vi "Main.vi"() -> ()   [LabVIEW 2018]
uses:
  <vilib>/addons/database/Connection.llb/DB Tools Open Connec (String).vi
  <vilib>/addons/database/NI_Database_API.lvlib
  <vilib>/ptbypt/NI_PtbyPt.lvlib
panel:
  out "100看门狗 2":i32
  in  "90数据":string[](array[string])
  in  "70数据":string[](array[string])
  out "Code":string
  in  "扫描到的条码":string
  in  "打印的条码":string
  out "退出":bool
  out "Main Tab":T1(tab)
  out "产品型号10":string
  out "产品型号20-90":string
  in  "其它信息":enum32{"信息", "错误信息"}(tab)
  out "ST20通讯状态":bool caption="ST30通讯状态"
  in  "ST100产品类型":string
  in  "ST100操作者":string
  in  "ST90产品类型":string
  in  "ST90操作者":string
  in  "ST80产品类型":string
  in  "ST80操作者":string
  in  "ST70产品类型":string
  in  "ST70操作者":string
  in  "ST60产品类型":string
  in  "ST60操作者":string
  in  "ST50产品类型":string
  in  "ST50操作者":string
  in  "ST40产品类型":string
  in  "ST40操作者":string
  in  "ST30产品类型":string
  in  "ST30操作者":string
  in  "ST20产品类型":string
  in  "ST20操作者":string
  in  "ST10产品类型":string
  in  "ST10操作者":string
  out "ST10通讯状态":bool
  out "ST30通讯状态":bool
  out "ST40通讯状态":bool caption="ST30通讯状态"
  out "ST70通讯状态":bool caption="ST30通讯状态"
  out "ST50通讯状态":bool caption="ST30通讯状态"
  out "ST60通讯状态":bool caption="ST30通讯状态"
  out "ST80通讯状态":bool caption="ST30通讯状态"
  out "ST90通讯状态":bool caption="ST30通讯状态"
  out "ST100通讯状态":bool caption="ST30通讯状态"
  in  "错误信息":i32(listbox)
  in  "每工站主要显示":T2(tab)
  in  "ST102_DATA":i32(listbox)=7 caption="ST10_DATA"
  in  "ST101_DATA":i32(listbox)=9 caption="ST10_DATA"
  out "ST10曲线":cluster{"X":dbl, "Y":dbl}[](graph) caption="ST20曲线"
  in  "选项卡控件":enum32{"数据", "曲线"}(tab)
  in  "ST202_DATA":i32(listbox) caption="ST20_DATA"
  in  "ST201_DATA":i32(listbox) caption="ST20_DATA"
  out "ST201_R曲线":cluster{"X":dbl, "Y":dbl}[](graph) caption="ST20曲线"
  out "ST202曲线":cluster{"X":dbl, "Y":dbl}[](graph) caption="ST20曲线"
  out "ST201_L曲线":cluster{"X":dbl, "Y":dbl}[](graph) caption="ST20曲线"
  in  "ST303_DATA":i32(listbox) caption="ST30_DATA"
  in  "ST302_DATA":i32(listbox) caption="ST30_DATA"
  in  "ST301_DATA":i32(listbox) caption="ST30_DATA"
  in  "ST402_DATA":i32(listbox) caption="ST40_DATA"
  in  "ST401_DATA":i32(listbox) caption="ST40_DATA"
  in  "选项卡控件 2":enum32{"数据1", "数据2", "曲线"}(tab)
  in  "ST502_DATA":i32(listbox)=4 caption="ST50_DATA"
  in  "ST501_DATA":i32(listbox)=4 caption="ST50_DATA"
  in  "ST504_DATA":i32(listbox)=4 caption="ST50_DATA"
  in  "ST503_DATA":i32(listbox)=4 caption="ST50_DATA"
  out "ST50_R曲线":cluster{"X":dbl, "Y":dbl}[](graph) caption="ST20曲线"
  out "ST50_L曲线":cluster{"X":dbl, "Y":dbl}[](graph) caption="ST20曲线"
  in  "ST603_DATA":i32(listbox) caption="ST60_DATA"
  in  "ST602_DATA":i32(listbox) caption="ST60_DATA"
  in  "ST601_DATA":i32(listbox) caption="ST60_DATA"
  in  "选项卡控件 3":enum32{"数据", "曲线"}(tab)
  in  "ST70_DATA":i32(listbox)=2
  out "ST70_R曲线":cluster{"X":dbl, "Y":dbl}[](graph) caption="ST20曲线"
  out "ST70_L曲线":cluster{"X":dbl, "Y":dbl}[](graph) caption="ST20曲线"
  in  "ST80_DATA":i32(listbox)
  in  "ST901_DATA":i32(listbox) caption="ST80_DATA"
  in  "ST902_DATA":i32(listbox) caption="ST80_DATA"
  in  "登录界面":bool
  in  "注销":bool
  in  "修改密码":bool
  in  "Rework界面":bool
  in  "界面切换":bool
  in  "登录界面返回":bool
  out "登录状态":string
  in  "登录":bool
  in  "输入管理员密码":string
  in  "修改密码界面返回":bool
  out "修改密码状态":string
  in  "确认修改密码":bool
  in  "新密码":string
  in  "初始密码":string
  in  "603":bool
  in  "602":bool
  in  "504":bool
  in  "402":bool
  in  "303":bool
  in  "302":bool
  in  "202":bool
  out "Rework状态":string
  in  "查询":bool
  in  "确定Rework":bool
  in  "Rework返回":bool
  in  "输入需要Rework的一维码：":string
  in  "102":bool
  in  "201":bool
  in  "301":bool
  in  "401":bool
  in  "501":bool
  in  "502":bool
  in  "503":bool
  in  "601":bool
  in  "70":bool
  in  "80":bool
  in  "901":bool
  in  "902":bool
  in  "Monitor Tab":T3(tab)
  out "产品型号":u32
  out "画曲线T-201 2":u32
  out "ST201文件移动中":bool caption="ST201保存中"
  out "ST201保存中":bool
  out "ST10画曲线":bool
  in  "303数据回复输入":bool
  in  "303扫码回复输入":bool
  out "数据保存请求回复303":string
  out "上一站号 (303)":string
  out "上一站结果 (303)":string
  out "扫码请求回复303":string
  out "303二维码":string
  out "ST303数据读取":bool
  out "ST303扫码请求":bool
  out "ST303数据读取 (事件)":bool
  out "ST303扫码请求 (事件)":bool
  in  "302数据回复输入":bool
  in  "302扫码回复输入":bool
  out "数据保存请求回复302":string
  out "上一站号 (302)":string
  out "上一站结果 (302)":string
  out "扫码请求回复302":string
  out "302二维码":string
  out "ST302数据读取":bool
  out "ST302扫码请求":bool
  out "ST302数据读取 (事件)":bool
  out "ST302扫码请求 (事件)":bool
  in  "301数据回复输入":bool
  in  "301扫码回复输入":bool
  out "ST202数据保存请求":bool
  out "ST202扫码请求":bool
  out "ST201数据保存请求":bool
  out "上一站结果 (202)":string
  out "上一站号 (202)":string
  in  "102数据回复写入":bool
  in  "102扫码回复写入":bool
  out "ST202扫码请求(事件)":bool
  out "ST202画曲线":bool
  out "ST202数据读取(事件)":bool
  out "ST201画曲线":bool
  out "ST201数据读取(事件)":bool
  out "ST201扫码请求(事件)":bool
  out "数据保存请求回复102":string
  out "扫码请求回复102":string
  out "上一站结果(10)":string
  out "上一站号(10)":string
  out "ST102扫码请求":bool
  out "ST101扫码请求":bool
  out "ST102数据读取":bool
  out "扫码请求回复101":string
  out "ST102扫码请求（事件）":bool
  out "ST101扫码请求（事件）":bool
  out "ST102数据读取（事件）":bool
  out "101二维码":string caption="101 二维码"
  out "ST201扫码请求":bool
  out "数据保存请求回复201":string
  out "扫码请求回复201":string
  out "上一站结果 (201)":string
  out "上一站号 (201)":string
  out "201二维码":string
  in  "返回":bool
  out "Sleeve_5020001":string
  out "20看门狗":i32
  out "10看门狗":i32
  out "Flange_5025570":string
  out "202二维码":string
  out "扫码请求回复202":string
  out "101打码等级":string
  out "102二维码":string caption="102 二维码"
  out "ST102数据":string[](array[string])
  in  "101扫码回复写入":bool
  in  "201扫码回复写入":bool
  in  "202扫码回复写入":bool
  in  "202数据回复写入":bool
  out "数据保存请求回复202":string
  in  "201数据回复写入":bool
  out "201数据":string[](array[string])
  out "202data":string[](array[string])
  out "30看门狗":i32
  out "数据保存请求回复301":string
  out "上一站号 (301)":string
  out "上一站结果 (301)":string
  out "扫码请求回复301":string
  out "301二维码":string
  out "ST301数据读取":bool
  out "ST301扫码请求":bool
  out "ST301数据读取 (事件)":bool
  out "ST301扫码请求 (事件)":bool
  out "301数据":string[](array[string])
  out "302data":string[](array[string])
  out "303data":string[](array[string])
  out "OP201文件?":bool
  out "画曲线T--201":u32
  out "打开时间":u32
  out "ST502画曲线":bool
  out "504data":string[](array[string])
  out "上一站号 (504)":string
  out "上一站结果 (504)":string
  out "数据保存请求回复504":string
  out "扫码请求回复504":string
  out "ST504数据读取（事件）":bool
  out "ST504扫码请求（事件）":bool
  out "ST504数据读取":bool
  out "ST504扫码请求":bool
  out "504二维码":string
  in  "504数据回复输入":bool
  in  "504扫码回复输入":bool
  out "上一站号 (503)":string
  out "上一站结果 (503)":string
  out "数据保存请求回复503":string
  out "扫码请求回复503":string
  out "ST503数据读取（事件）":bool
  out "ST503扫码请求（事件）":bool
  out "上一站号 (502)":string
  out "上一站结果 (502)":string
  out "数据保存请求回复502":string
  out "扫码请求回复502":string
  out "ST502数据读取（事件）":bool
  out "ST502扫码请求（事件）":bool
  out "上一站号 (501)":string
  out "上一站结果 (501)":string
  out "数据保存请求回复501":string
  out "扫码请求回复501":string
  out "ST501数据读取（事件）":bool
  out "ST501扫码请求（事件）":bool
  out "ST401数据保存请求":bool
  out "ST401扫码请求":bool
  out "ST401数据读取（事件）":bool caption="ST401数据保存请求（事件）"
  out "ST401扫码请求（事件）":bool
  out "数据保存请求回复401":string
  out "扫码请求回复401":string
  out "401二维码":string
  in  "401数据回复写入":bool
  in  "401扫码回复写入":bool
  out "上一站号 (401)":string
  out "上一站结果 (401)":string
  out "ST402数据保存请求":bool
  out "ST402扫码请求":bool
  out "402data":string[](array[string])
  out "402二维码":string
  out "401数据":string[](array[string])
  out "40看门狗":i32
  in  "402扫码回复写入":bool
  in  "402数据回复写入":bool
  out "ST402数据读取（事件）":bool caption="ST402数据保存请求（事件）"
  out "ST402扫码请求（事件）":bool
  out "上一站号 (402)":string
  out "上一站结果 (402)":string
  out "数据保存请求回复402":string
  out "扫码请求回复402":string
  out "503data":string[](array[string])
  out "503二维码":string
  out "ST503数据读取":bool
  out "ST503扫码请求":bool
  out "ST502数据读取":bool
  out "ST502扫码请求":bool
  out "ST501数据读取":bool
  out "ST501扫码请求":bool
  out "502二维码":string
  out "501二维码":string
  in  "503数据回复输入":bool
  in  "503扫码回复输入":bool
  in  "502数据回复输入":bool
  in  "502扫码回复输入":bool
  in  "501数据回复输入":bool
  in  "501扫码回复输入":bool
  out "50看门狗":i32
  out "501data":string[](array[string])
  out "502数据":string[](array[string])
  out "ST70画曲线":bool
  out "上一站结果 (80)":string
  out "上一站号 (80)":string
  out "扫码请求回复80":string
  out "数据保存请求回复80":string
  out "ST80数据保存请求（事件）":bool
  out "ST80扫码请求 （事件）":bool caption="ST80扫码请求（事件）"
  out "数据保存请求回复70":string
  out "ST70数据读取（事件）":bool caption="ST70数据读取(事件)"
  out "上一站结果 (603)":string
  out "上一站号 (603)":string
  out "扫码请求回复603":string
  out "数据保存请求回复603":string
  out "ST603数据读取（事件）":bool
  out "ST603扫码请求（事件）":bool
  out "上一站结果 (602)":string
  out "上一站号 (602)":string
  out "扫码请求回复602":string
  out "数据保存请求回复602":string
  out "ST602数据读取（事件）":bool
  out "ST602扫码请求 （事件）":bool caption="ST602扫码请求（事件）"
  out "ST601数据读取（事件）":bool
  out "ST601扫码请求（事件）":bool
  out "603data":string[](array[string])
  out "603二维码":string
  out "ST603数据读取":bool
  out "ST603扫码请求":bool
  out "ST602数据读取":bool
  out "ST602扫码请求":bool
  out "ST601数据读取":bool
  out "ST601扫码请求":bool
  out "602data":string[](array[string])
  out "602二维码":string
  out "601数据":string[](array[string])
  out "601二维码":string
  in  "603数据回复输入":bool
  in  "603扫码回复输入":bool
  in  "602数据回复输入":bool
  in  "602扫码回复输入":bool
  in  "601数据回复输入":bool
  in  "601扫码回复输入":bool
  out "60看门狗":i32
  out "扫码请求回复601":string
  out "数据保存请求回复601":string
  out "上一站结果 (601)":string
  out "上一站号 (601)":string
  out "ST70数据读取":bool
  out "70编码":string
  in  "70数据回复输入":bool
  out "70看门狗":i32
  out "70数据":string[](array[string])
  out "ST70_Housing_5025351":string
  out "ST70_Bushing_5025400":string
  out "ST80数据保存请求":bool
  out "ST80扫码请求":bool
  out "80二维码":string
  in  "80数据回复写入":bool
  in  "80扫码回复写入":bool
  out "ST80_Spring_5024883":string
  out "ST80_Flat_sael_5020064":string
  out "ST80_Spring_plate_5025473":string
  out "80看门狗":i32
  out "80数据":string[](array[string])
  in  "ST70数据读取（事件） 2":bool caption="ST70数据读取(手动事件)"
  in  "70数据 2-手动测试":string[](array[string])
  out "ST90画曲线":bool
  in  "901数据回复输入":bool
  out "上一站号 (901)":string
  out "上一站结果 (901)":string
  out "数据保存请求回复901":string
  out "扫码请求回复901":string
  in  "901扫码回复输入":bool
  out "901二维码":string
  out "ST901扫码请求":bool
  out "ST901数据读取":bool
  out "ST901扫码请求（事件）":bool
  out "ST901数据读取（事件）":bool
  in  "901编码回复输入":bool
  out "901编码":string
  out "ST901编码请求":bool
  out "ST901编码请求 （事件）":bool caption="ST901编码请求（事件）"
  out "编码请求回复901":string
  out "上一站号 (901) 编码":string caption="上一站号 (901编码)"
  out "上一站结果 (901)编码":string caption="上一站结果 (901编码)"
  in  "902扫码回复输入":bool
  in  "902数据回复输入":bool
  out "ST902扫码请求":bool
  out "ST902数据读取":bool
  out "902二维码":string
  out "ST902扫码请求（事件）":bool
  out "ST902数据读取（事件）":bool
  out "数据保存请求回复902":string
  out "扫码请求回复902":string
  out "上一站号 (902)":string
  out "上一站结果 (902)":string
  out "901数据":string[](array[string])
  out "902数据":string[](array[string])
  out "90看门狗":i32
  out "ST100扫码请求":bool
  out "ST100扫码请求（事件）":bool
  out "上一站结果 (100)":string
  out "上一站号 (100)":string
  out "100二维码":string
  in  "100扫码回复输入":bool
  out "100看门狗":i32
  out "扫码请求回复100":string
  out "压机旋铆位移压力图_4":cluster{dbl[], dbl[]}(graph)
  out "压机旋铆位移压力图_3":cluster{dbl[], dbl[]}(graph)
  out "压机旋铆位移压力图_2":cluster{dbl[], dbl[]}(graph)
  out "压机旋铆位移压力图_1":cluster{dbl[], dbl[]}(graph)
  out "压机旋铆位移压力图_5":cluster{dbl[], dbl[]}(graph)
  # "V1.0"
  # "数据库追溯系统"
  # "v3.0"
  # "登 录"
  # "修 改 密 码"
  # "ST30"
  # "ST10"
  # "ST20"
  # "ST60"
  # "ST70"
  # "ST80"
  # "ST100"
  # "ST90"
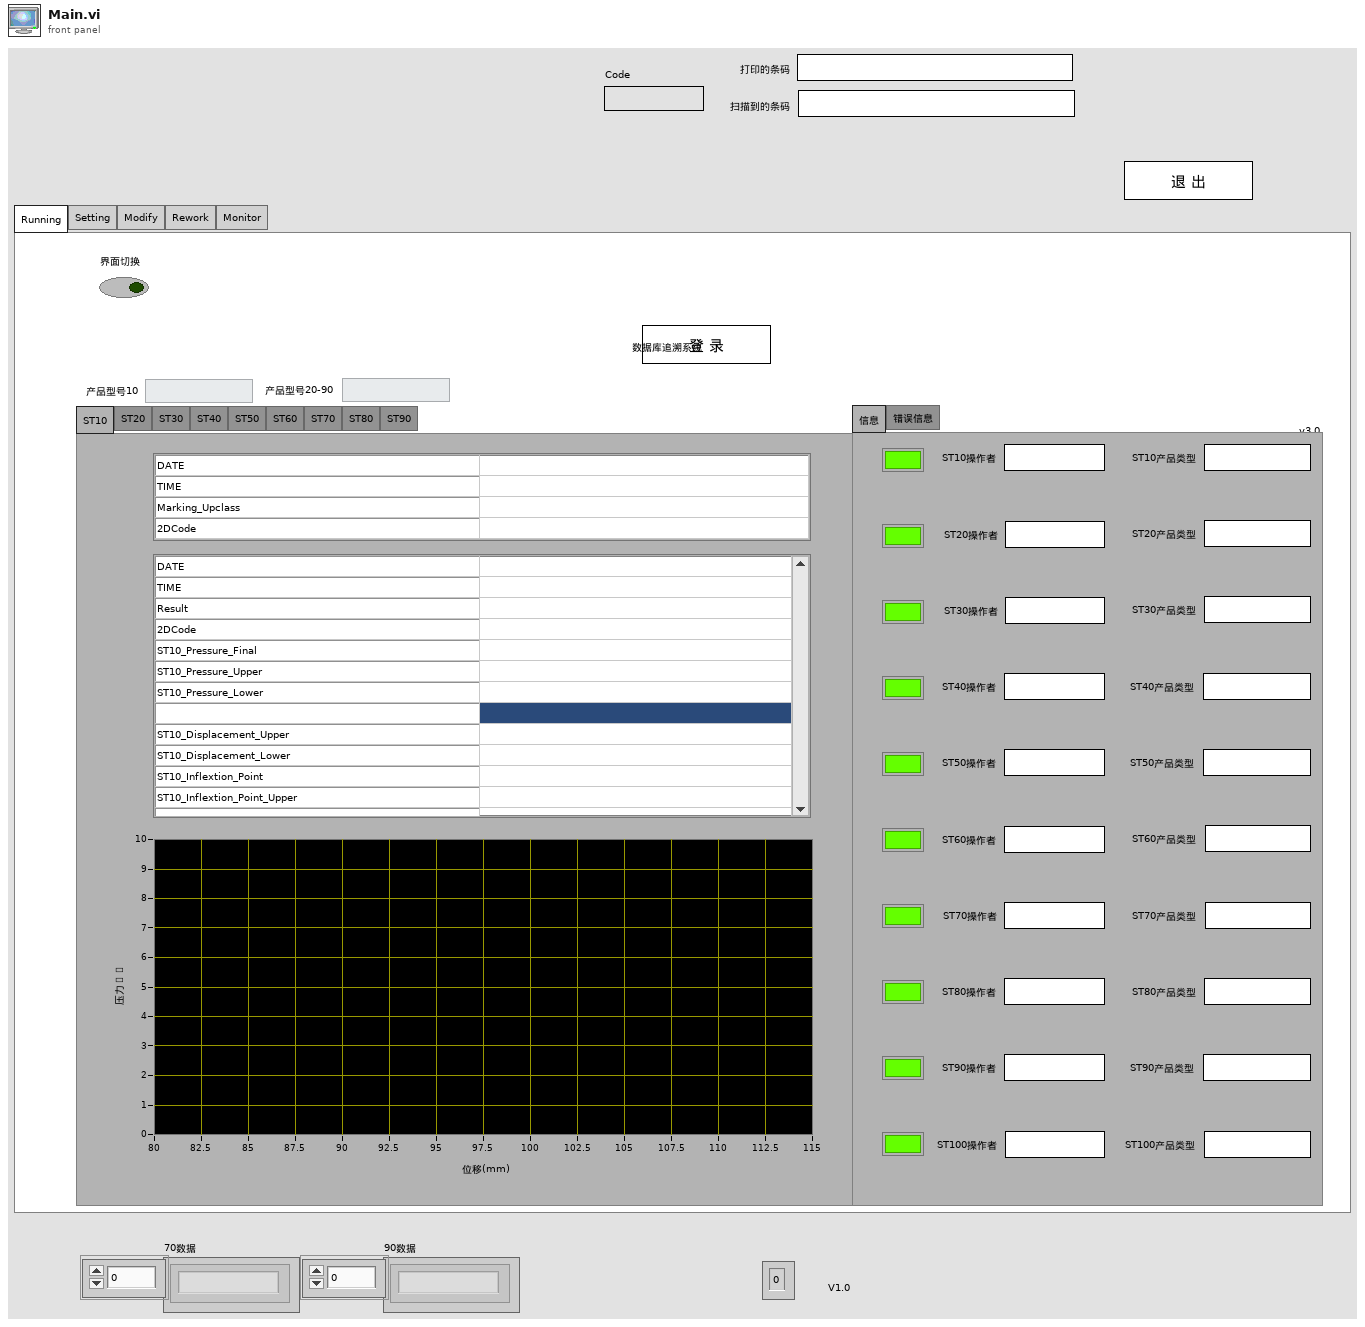
[diagram p1: front panel]
types:
  T1 = enum32{"Running", "Setting", "Modify", "Rework", "Monitor"}
  T2 = enum32{"ST10", "ST20", "ST30", "ST40", "ST50", "ST60", "ST70", "ST80", "ST90"}
  T3 = enum32{"Interface 1", "Interface 2", "Interface 3", "Interface 4", "Interface 7", "Interface 8"}
  T4 = enum32{"Invalid", "Standard", "Closed", "Hidden", "Minimized", "Maximized"}
  T5 = typedef "NI_Database_API.lvlib/Conn ObjectReference.ctl" = refnum<k1>
diagram:
  n1 = flat-sequence {
    tunnel: [w9] -> w2
    tunnel: [w8] -> w1
    tunnel: w2 -> [w35]
    tunnel: w1 -> [w36]
    frame #0 {
      w6 = "Code" ("subkeyName")
      w4 = FALSE ("可见")
      n2 = call "Read Registry.vi"("value"=w6, "subkeyName"=w6) -> ("Data"=→"Code":string)  [unwired: 6 in, 1 out]
      n3 = property on="Rework界面" class="Bool"("Visible"=w4) -> ()  [unwired: 2 in, 2 out]
      n4 = property on="注销" class="Bool"("Visible"=w4) -> ()  [unwired: 2 in, 2 out]
      n5 = property on="修改密码" class="Bool"("Visible"=w4) -> ()  [unwired: 2 in, 2 out]
      n6 = property on="界面切换" class="Bool (严格)"("Visible"=FALSE ("可见")) -> ()  [unwired: 2 in, 2 out]
      n7 = call-poly <vilib>:"DB Tools Open Connection.vi"("connection information"="DQ501") -> ("error out"=w8:errorcluster, "connection reference"=w9:T5)  [unwired: 7 in]
    }
    frame #1 {
      # "10\n201\n202\n50\n70"
      # "字符串的初始地址都加2位"
      # "报警日志 ：Alarm_Log\n历史程序：History program\n数据保存：data storage\n曲线curve\n数据data"
      # "报警日志 ：Alarm_Log\n历史程序：History program\n数据保存：data storage\n曲线curve\n数据data"
      # "报警日志 ：Alarm_Log\n历史程序：History program\n数据保存：data storage\n曲线curve\n数据data"
      # "报警日志 ：Alarm_Log\n历史程序：History program\n数据保存：data storage\n曲线curve\n数据data"
      # "报警日志 ：Alarm_Log\n历史程序：History program\n数据保存：data storage\n曲线curve\n数据data"
      # "对数据库操作的事件"
      # "其余事件 如曲线保存"
      n8 = constructor class="CloseExcel"() -> (reference out=w14:refnum<k24>, error out=w12:errorcluster)  [unwired: 3 in, 1 out]
      n9 = invoke class="CloseExcel" method="OpenProgram"(reference=w14, error in=w12) -> (reference out=w13:refnum<k24>, error out=w11:errorcluster)  [unwired: 1 in, 1 out]
      n10 = case shown="错误" w11 {
        selector: w11 -> [_ w40]
        tunnel: "CloseExcel进程打开失败！" -> [_ w43]
        frame No Error {
        }
        frame Error {
          n11 = property on="错误信息" class="LstBox (严格)"() -> ("Item Names"=w38:string[])  [unwired: 2 in, 2 out]
          n12 = Unbundle By Name(w40) -> ("source"=w39:string)
          n13 = Format Date/Time String(time format string (%c)="%Y-%m-%d %H:%M:%S" ("时间格式字符串(%c)")) -> (date/time string=w45:string)  [unwired: 2 in]
          n14 = Concatenate Strings(w45, "  " ("字符串"), w43, w39) -> (w41:string)
          n15 = Insert Into Array(array=w38, index=0 ("索引"), new element=w41) -> (w37:string[])
          n16 = property on="错误信息" class="LstBox (严格)"("Item Names"=w37) -> ()  [unwired: 2 in, 2 out]
        }
      }
      n17 = while {
        tunnel: w36 -> [w7757]
        tunnel: w35 -> [w7756]
        tunnel: w13 -> [w7755]
        stop <- w7759 stop-if-true
        n18 = event shown="[9] \"注销\": 值改变" {
          selector: _ -> [_ _ _ _ _ _ _ _ _ _ _ _ _ _ _ _ _ _]
          dyn-events: _ -> [_ _ _ _ _ _ _ _ _ _ _ _ _ _ _ _ _ _]
          timeout: 10 -> [_ _ _ _ _ _ _ _ _ _ _ _ _ _ _ _ _ _]
          tunnel: [FALSE TRUE FALSE FALSE FALSE FALSE FALSE FALSE FALSE FALSE FALSE FALSE FALSE FALSE _ FALSE _ _] -> w7759
          tunnel: w7757 -> [_ w7766 _ _ _ _ _ _ _ _ _ _ _ _ _ _ _ _]
          tunnel: w7756 -> [_ w7765 _ _ _ _ _ _ _ _ _ _ _ _ _ _ _ _]
          tunnel: w7755 -> [_ w7762 _ _ _ _ _ _ _ _ _ _ _ _ _ _ _ _]
          event Timeout {
            n19 = event-data() -> ()  [unwired: 1 in, 3 out]
          }
          event Panel Close {
            n20 = event-data() -> ()  [unwired: 1 in, 3 out]
            n21 = invoke class="CloseExcel" method="CloseProgram"(reference=w7762) -> ()  [unwired: 2 in, 3 out]
            n22 = call <vilib>:"DB Tools Close Connection.vi"("error in (no error)"=w7766, "connection reference"=w7765) -> ()  [unwired: 5 in, 1 out]
            n23 = flat-sequence {
              frame #0 {
                n24 = property on="错误信息" class="LstBox (严格)"() -> ("Item Names"=w7769:string[])  [unwired: 2 in, 2 out]
                n25 = Array Size(array=w7769) -> (size(s)=w7768:i32)
                n26 = Equal To 0?(x=w7768) -> (x = 0?=w7767:bool)
                n27 = case shown="假" w7767 {
                  tunnel: w7769 -> [w7770 _]
                  frame False {
                    n28 = call <vilib>:"Check if File or Folder Exists.vi"("path"=path "D:/Alarm_Log") -> ("error out"=w7786:errorcluster, "file or folder exists?"=w7787:bool, "dup path"=w7785:path)  [unwired: 8 in]
                    n29 = Format Date/Time String(time format string (%c)="%Y%m%d" ("时间格式字符串(%c)")) -> (date/time string=w7782:string)  [unwired: 2 in]
                    n30 = case shown="真" w7787 {
                      tunnel: w7786 -> [w7802 w7803]
                      tunnel: w7785 -> [w7801 w7804]
                      tunnel: [w7800 w7804] -> w7784
                      tunnel: [w7799 w7803] -> w7779
                      frame False {
                        n31 = Create Folder(path (use dialog)=w7801, error in=w7802) -> (created path=w7800:path, error out=w7799:errorcluster)  [unwired: 1 in, 1 out]
                      }
                      frame True {
                      }
                    }
                    n32 = Concatenate Strings(w7782, ".txt" ("字符串")) -> (w7780:string)
                    n33 = Build Path(base path=w7784, name or relative path=w7780) -> (appended path=w7773:path)
                    n34 = call <vilib>:"Check if File or Folder Exists.vi"("error in (no error)"=w7779, "path"=w7773) -> ("error out"=w7777:errorcluster, "file or folder exists?"=w7778:bool, "dup path"=w7776:path)  [unwired: 7 in]
                    n35 = case shown="假" w7778 {
                      tunnel: w7777 -> [_ w7792]
                      tunnel: w7776 -> [_ w7791]
                      tunnel: [string[] [] ("array of strings") w7790] -> w7774
                      frame False {
                      }
                      frame True {
                        n36 = Read from Text File(file (use dialog)=w7791, error in=w7792) -> (text=w7793:string)  [unwired: 2 in, 3 out]
                        n37 = Search and Replace String(replace all?=TRUE ("替换全部？(F)"), input string=w7793, search string="\n" ("搜索字符串"), replace string="\\" ("替换字符串(\"\")")) -> (result string=w7797:string)  [unwired: 4 in, 3 out]
                        n38 = String To Path(string=w7797) -> (path=w7798:path)
                        n39 = Path to Array of Strings(0:w7798) -> (2:w7790:string[])  [unwired: 1 out]
                      }
                    }
                    n40 = Array Size(array=w7770) -> (size(s)=w7775:i32)
                    n41 = Insert Into Array(array=w7770, index=w7775, new element=w7774) -> (w7772:string[])
                    n42 = Write to Text File(file (use dialog)=w7773, text=w7772) -> (error out=w7771:errorcluster)  [unwired: 2 in, 2 out]
                    n43 = call <vilib>:"Clear Errors.vi"("error in (no error)"=w7771) -> ()  [unwired: 5 in, 2 out]
                  }
                  frame True {
                  }
                }
              }
              frame #1 {
                n44 = control-ref of="本VI"() -> (w7805:refnum<vi>)
                n45 = property class="VI"(reference=w7805, "FP.State"=T4."Closed" ("前面板窗口:状态")) -> ()  [unwired: 1 in, 2 out]
              }
            }
            "退出" <- TRUE ("退出")
          }
          event "界面切换": Value Change {
            n46 = event-data() -> ()  [unwired: 1 in, 3 out]
            "Main Tab" <- T1."Monitor" ("Main Tab")
          }
          event "返回": Value Change {
            n47 = event-data() -> ()  [unwired: 1 in, 3 out]
            n48 = local write "Main Tab"(T1."Running" ("Main Tab")) -> ()
          }
          event "登录界面": Value Change {
            w7811 = "" ("输入管理员密码")
            n49 = event-data() -> ()  [unwired: 1 in, 3 out]
            n50 = local write "登录状态"(w7811) -> ()
            n51 = local write "输入管理员密码"(w7811) -> ()
            n52 = local write "Main Tab"(T1."Setting" ("Main Tab")) -> ()
          }
          event "登录": Value Change {
            n53 = event-data() -> ()  [unwired: 1 in, 3 out]
            n54 = Equal?(x="输入管理员密码", y="18202173350") -> (x = y?=w7814:bool)
            n55 = case shown="真" w7814 {
              tunnel: "输入管理员密码" -> [w7825 _]
              tunnel: [w7824 TRUE] -> w7815
              frame False {
                n56 = local read "Code"() -> (w7826:string)
                n57 = Equal?(x=w7825, y=w7826) -> (x = y?=w7824:bool)
              }
              frame True {
                n58 = property on="界面切换" class="Bool (严格)"("Visible"=TRUE ("可见")) -> ()  [unwired: 2 in, 2 out]
              }
            }
            n59 = case shown="真" w7815 {
              tunnel: ["登录失败！" ("登录状态") "登录成功！" ("登录状态")] -> w7816
              frame False {
              }
              frame True {
                w7822 = TRUE ("可见")
                n60 = property on="修改密码" class="Bool"("Visible"=w7822) -> ()  [unwired: 2 in, 2 out]
                n61 = property on="Rework界面" class="Bool"("Visible"=w7822) -> ()  [unwired: 2 in, 2 out]
                n62 = property on="注销" class="Bool"("Visible"=w7822) -> ()  [unwired: 2 in, 2 out]
                n63 = local write "Main Tab"(T1."Running" ("Main Tab")) -> ()
              }
            }
            "登录状态" <- w7816
          }
          event "修改密码界面返回", "登录界面返回", "Rework返回": Value Change {
            n64 = event-data() -> ()  [unwired: 1 in, 3 out]
            n65 = local write "Main Tab"(T1."Running" ("Main Tab")) -> ()
          }
          event "Rework界面": Value Change {
            w7831 = FALSE ("503")
            w7834 = "" ("输入需要Rework的一维码：")
            n66 = event-data() -> ()  [unwired: 1 in, 3 out]
            n67 = local write "603"(w7831) -> ()
            n68 = local write "602"(w7831) -> ()
            n69 = local write "504"(w7831) -> ()
            n70 = local write "402"(w7831) -> ()
            n71 = local write "303"(w7831) -> ()
            n72 = local write "302"(w7831) -> ()
            n73 = local write "202"(w7831) -> ()
            n74 = local write "102"(w7831) -> ()
            n75 = local write "503"(w7831) -> ()
            n76 = local write "601"(w7831) -> ()
            n77 = local write "70"(w7831) -> ()
            n78 = local write "80"(w7831) -> ()
            n79 = local write "901"(w7831) -> ()
            n80 = local write "902"(w7831) -> ()
            n81 = local write "201"(w7831) -> ()
            n82 = local write "301"(w7831) -> ()
            n83 = local write "401"(w7831) -> ()
            n84 = local write "501"(w7831) -> ()
            n85 = local write "502"(w7831) -> ()
            n86 = local write "Rework状态"(w7834) -> ()
            n87 = local write "输入需要Rework的一维码："(w7834) -> ()
            n88 = local write "Main Tab"(T1."Rework" ("Main Tab")) -> ()
          }
          event "102", "201", "202", "301", "302", "303", "401", "402", "501", "502", "503", "504", "601", "602", "603", "70", "80", "901", "902": Value Change {
            w7835 = cluster{u32, u32}[] [{1985280, 1985280}, {6618880, 6618880}, {1985280, 1985280}, {6618880, 6618880}] ("颜色[4]")
            n89 = event-data() -> ()  [unwired: 1 in, 3 out]
            n90 = property on="102" class="Bool (严格)"("Colors [4]"=w7835) -> ()  [unwired: 2 in, 2 out]
            n91 = property on="201" class="Bool (严格)"("Colors [4]"=w7835) -> ()  [unwired: 2 in, 2 out]
            n92 = property on="301" class="Bool (严格)"("Colors [4]"=w7835) -> ()  [unwired: 2 in, 2 out]
            n93 = property on="401" class="Bool (严格)"("Colors [4]"=w7835) -> ()  [unwired: 2 in, 2 out]
            n94 = property on="501" class="Bool (严格)"("Colors [4]"=w7835) -> ()  [unwired: 2 in, 2 out]
            n95 = property on="502" class="Bool (严格)"("Colors [4]"=w7835) -> ()  [unwired: 2 in, 2 out]
            n96 = property on="503" class="Bool (严格)"("Colors [4]"=w7835) -> ()  [unwired: 2 in, 2 out]
            n97 = property on="601" class="Bool (严格)"("Colors [4]"=w7835) -> ()  [unwired: 2 in, 2 out]
            n98 = property on="70" class="Bool (严格)"("Colors [4]"=w7835) -> ()  [unwired: 2 in, 2 out]
            n99 = property on="80" class="Bool (严格)"("Colors [4]"=w7835) -> ()  [unwired: 2 in, 2 out]
            n100 = property on="901" class="Bool (严格)"("Colors [4]"=w7835) -> ()  [unwired: 2 in, 2 out]
            n101 = property on="902" class="Bool (严格)"("Colors [4]"=w7835) -> ()  [unwired: 2 in, 2 out]
            n102 = property on="602" class="Bool (严格)"("Colors [4]"=w7835) -> ()  [unwired: 2 in, 2 out]
            n103 = property on="603" class="Bool (严格)"("Colors [4]"=w7835) -> ()  [unwired: 2 in, 2 out]
            n104 = property on="202" class="Bool (严格)"("Colors [4]"=w7835) -> ()  [unwired: 2 in, 2 out]
            n105 = property on="302" class="Bool (严格)"("Colors [4]"=w7835) -> ()  [unwired: 2 in, 2 out]
            n106 = property on="303" class="Bool (严格)"("Colors [4]"=w7835) -> ()  [unwired: 2 in, 2 out]
            n107 = property on="402" class="Bool (严格)"("Colors [4]"=w7835) -> ()  [unwired: 2 in, 2 out]
            n108 = property on="504" class="Bool (严格)"("Colors [4]"=w7835) -> ()  [unwired: 2 in, 2 out]
          }
          event "注销": Value Change {
            w7838 = FALSE ("可见")
            n109 = event-data() -> ()  [unwired: 1 in, 3 out]
            n110 = property on="界面切换" class="Bool (严格)"("Visible"=FALSE ("可见")) -> ()  [unwired: 2 in, 2 out]
            n111 = property on="Rework界面" class="Bool"("Visible"=w7838) -> ()  [unwired: 2 in, 2 out]
            n112 = property on="修改密码" class="Bool"("Visible"=w7838) -> ()  [unwired: 2 in, 2 out]
            n113 = property on="注销" class="Bool"("Visible"=w7838) -> ()  [unwired: 2 in, 2 out]
          }
          event "修改密码": Value Change {
            w7840 = "" ("修改密码状态")
            n114 = event-data() -> ()  [unwired: 1 in, 3 out]
            n115 = local write "Main Tab"(T1."Modify" ("Main Tab")) -> ()
            n116 = local write "修改密码状态"(w7840) -> ()
            n117 = local write "新密码"(w7840) -> ()
            n118 = local write "初始密码"(w7840) -> ()
          }
          event "确认修改密码": Value Change {
            n119 = event-data() -> ()  [unwired: 1 in, 3 out]
            n120 = local read "Code"() -> (w7845:string)
            n121 = Equal?(x="初始密码", y=w7845) -> (x = y?=w7844:bool)
            n122 = case shown="真" w7844 {
              tunnel: ["初始密码错误" ("修改密码状态") w7850] -> w7843
              frame False {
              }
              frame True {
                w7852 = "Code" ("subkeyName")
                n123 = call "Write Registry.vi"("value"=w7852, "data"="新密码", "subkeyName"=w7852) -> ("error out"=w7851:errorcluster)  [unwired: 8 in]
                n124 = case shown="无错误" w7851 {
                  tunnel: ["修改密码成功" ("修改密码状态") "修改密码失败" ("修改密码状态")] -> w7850
                  tunnel: "新密码" -> [w7853 _]
                  frame No Error {
                    n125 = local write "Code"(w7853) -> ()
                  }
                  frame Error {
                  }
                }
              }
            }
            "修改密码状态" <- w7843
          }
          event "ST10画曲线": Value Change {
            n126 = event-data() -> ()  [unwired: 1 in, 3 out]
            n127 = call "检查曲线文件.vi"("Folder Path"=path "D:/op10" ("路径")) -> ("Error Out"=w7859:errorcluster, "Exit?"=w7861:bool, "曲线文件路径"=w7860:path)  [unwired: 7 in, 1 out]
            n128 = case shown="真" w7861 {
              tunnel: w7860 -> [_ w7883]
              tunnel: w7859 -> [w7879 w7882]
              tunnel: [w7879 w7881] -> w7858
              frame False {
              }
              frame True {
                n129 = flat-sequence {
                  tunnel: [w7886] -> w7884
                  tunnel: w7883 -> [w7885]
                  tunnel: w7882 -> [w7887]
                  tunnel: [w7885] -> w7880
                  tunnel: w7884 -> [w7913]
                  tunnel: [w7903] -> w7881
                  tunnel: w7880 -> [w7894]
                  frame #0 {
                    n130 = call "EXCEL 画曲线.vi"("错误输入（无错误）"=w7887, "路径"=w7885) -> ("error IO"=w7886:errorcluster, "XY图"=→"ST10曲线":cluster{"X":dbl, "Y":dbl}[])  [unwired: 6 in, 2 out]
                  }
                  frame #1 {
                    n131 = local read "101二维码"() -> (w7889:string)
                    n132 = call "图片保存.vi"("一维码"=w7889) -> ("dup path"=w7904:path)  [unwired: 9 in, 1 out]
                    n133 = Build Path(base path=w7904, name or relative path=w7889) -> (appended path=w7905:path)
                    n134 = call <vilib>:"Check if File or Folder Exists.vi"("path"=w7905) -> ("error out"=w7907:errorcluster, "file or folder exists?"=w7906:bool)  [unwired: 8 in, 1 out]
                    n135 = case shown="假" w7906 {
                      tunnel: w7905 -> [w7924 w7926]
                      tunnel: [w7923 w7926] -> w7897
                      tunnel: w7907 -> [w7922 w7925]
                      tunnel: [w7921 w7925] -> w7898
                      frame False {
                        n136 = Create Folder(path (use dialog)=w7924, error in=w7922) -> (created path=w7923:path, error out=w7921:errorcluster)  [unwired: 1 in, 1 out]
                      }
                      frame True {
                      }
                    }
                    n137 = Concatenate Strings(w7889, "ST10.BMP" ("字符串")) -> (w7910:string)
                    n138 = Build Path(base path=w7897, name or relative path="ST10" ("名称或相对路径")) -> (appended path=w7899:path)
                    n139 = call <vilib>:"Check if File or Folder Exists.vi"("error in (no error)"=w7898, "path"=w7899) -> ("error out"=w7900:errorcluster, "file or folder exists?"=w7901:bool)  [unwired: 7 in, 1 out]
                    n140 = case shown="假" w7901 {
                      tunnel: w7899 -> [w7918 w7920]
                      tunnel: [w7917 w7920] -> w7893
                      tunnel: w7900 -> [w7916 w7919]
                      tunnel: [w7915 w7919] -> _
                      frame False {
                        n141 = Create Folder(path (use dialog)=w7918, error in=w7916) -> (created path=w7917:path, error out=w7915:errorcluster)  [unwired: 1 in, 1 out]
                      }
                      frame True {
                      }
                    }
                    n142 = Build Path(base path=w7893, name or relative path=w7910) -> (appended path=w7892:path)
                    n143 = call "文件路径.vi"("文件路径"=w7892, "文件格式"=".BMP") -> ("新路径"=w7891:path)  [unwired: 9 in]
                    n144 = invoke on="ST10曲线" class="XYGraph (严格)" method="Export Image"(error in=w7913, "FileType"=enum32{"BMP", "EPS", "EMF", "PICT"}."BMP" ("文件类型"), "Target"=enum32{"File", "Clipboard"}."File" ("目标"), "Path"=w7891, "HideGrid"=FALSE ("隐藏网格"), "Overwrite"=TRUE ("隐藏网格")) -> (error out=w7895:errorcluster)  [unwired: 2 in, 7 out]
                    n145 = Move(source path=w7894, error in=w7895, 9:TRUE ("覆盖(F)"), 10:w7893) -> (error out=w7903:errorcluster)  [unwired: 1 in, 2 out]
                  }
                }
              }
            }
            n146 = case shown="错误" w7858 {
              selector: w7858 -> [_ w7870]
              frame No Error {
                n147 = local write "102数据回复写入"(TRUE ("102数据回复写入")) -> ()
                n148 = local write "数据保存请求回复102"("1" ("数据保存请求回复102")) -> ()
              }
              frame Error {
                n149 = Unbundle By Name(w7870) -> ("source"=w7869:string)
                n150 = property on="错误信息" class="LstBox (严格)"() -> ("Item Names"=w7876:string[])  [unwired: 2 in, 2 out]
                n151 = Format Date/Time String(time format string (%c)="%Y-%m-%d %H:%M:%S" ("时间格式字符串(%c)")) -> (date/time string=w7871:string)  [unwired: 2 in]
                n152 = Concatenate Strings(w7871, "——" ("字符串"), w7869) -> (w7867:string)
                n153 = local write "102数据回复写入"(TRUE ("102数据回复写入")) -> ()
                n154 = local write "数据保存请求回复102"("2" ("数据保存请求回复102")) -> ()
                n155 = Concatenate Strings(w7867, "  " ("字符串"), "ST10 画曲线错误") -> (w7874:string)
                n156 = Insert Into Array(array=w7876, index=0 ("索引"), new element=w7874) -> (w7873:string[])
                n157 = property on="错误信息" class="LstBox (严格)"("Item Names"=w7873) -> ()  [unwired: 2 in, 2 out]
              }
            }
            "ST10画曲线" <- FALSE ("ST10画曲线")
          }
          event "ST201画曲线": Value Change {
            n158 = event-data() -> ()  [unwired: 1 in, 3 out]
            n159 = stacked-sequence {
              tunnel: [_ w7931 _ _] -> w7927
              frame #0 {
                "ST201文件移动中" <- TRUE ("ST201文件移动中")
              }
              frame #1 {
                n160 = call "检查曲线文件.vi"("Folder Path"=path "D:/op201" ("路径")) -> ("Error Out"=w7932:errorcluster, "Exit?"=w7934:bool, "曲线文件路径"=w7933:path)  [unwired: 7 in, 1 out]
                n161 = case shown="真" w7934 {
                  tunnel: w7933 -> [_ w7951]
                  tunnel: w7932 -> [w7936 w7950]
                  tunnel: [w7936 w7949] -> w7931
                  frame False {
                  }
                  frame True {
                    n162 = flat-sequence {
                      tunnel: w7950 -> [w7953]
                      tunnel: w7951 -> [w7954]
                      tunnel: [w7954] -> w7948
                      tunnel: [w7953] -> w7947
                      tunnel: [w7952] -> w7941
                      tunnel: [w7958] -> w7946
                      tunnel: [w7957] -> w7944
                      tunnel: w7948 -> [w7957]
                      tunnel: w7947 -> [w7959]
                      tunnel: [w7956] -> w7942
                      tunnel: w7941 -> [w7956]
                      tunnel: w7946 -> [w7964]
                      tunnel: [w7964] -> w7945
                      tunnel: w7944 -> [w7963]
                      tunnel: [w7963] -> w7943
                      tunnel: w7942 -> [w7961]
                      tunnel: [w7962] -> w7940
                      tunnel: [w7961] -> w7939
                      tunnel: w7945 -> [w7992]
                      tunnel: w7943 -> [w7973]
                      tunnel: w7940 -> [w7965]
                      tunnel: w7939 -> [w7967]
                      tunnel: [w7982] -> w7938
                      tunnel: [w7965] -> w7937
                      tunnel: [w8009] -> w7949
                      tunnel: w7938 -> [w8009]
                      tunnel: w7937 -> [w8007]
                      frame #0 {
                        n163 = Tick Count (ms)() -> (millisecond timer value=w7952:u32)
                      }
                      frame #1 {
                        n164 = call "EXCEL 画曲线.vi"("错误输入（无错误）"=w7959, "路径"=w7957) -> ("error IO"=w7958:errorcluster, "打开时间"=→"打开时间":u32, "XY图"=→"ST201_R曲线":cluster{"X":dbl, "Y":dbl}[])  [unwired: 6 in, 1 out]
                      }
                      frame #2 {
                        n165 = Tick Count (ms)() -> (millisecond timer value=w7962:u32)
                      }
                      frame #3 {
                        n166 = local read "201二维码"() -> (w7971:string)
                        n167 = Subtract(x=w7965, y=w7967) -> (x-y=→"画曲线T--201":u32)
                        n168 = call "图片保存.vi"("一维码"=w7971) -> ("dup path"=w7983:path)  [unwired: 9 in, 1 out]
                        n169 = Build Path(base path=w7983, name or relative path=w7971) -> (appended path=w7984:path)
                        n170 = call <vilib>:"Check if File or Folder Exists.vi"("path"=w7984) -> ("error out"=w7986:errorcluster, "file or folder exists?"=w7985:bool)  [unwired: 8 in, 1 out]
                        n171 = case shown="假" w7985 {
                          tunnel: w7984 -> [w8003 w8005]
                          tunnel: [w8002 w8005] -> w7976
                          tunnel: w7986 -> [w8001 w8004]
                          tunnel: [w8000 w8004] -> w7977
                          frame False {
                            n172 = Create Folder(path (use dialog)=w8003, error in=w8001) -> (created path=w8002:path, error out=w8000:errorcluster)  [unwired: 1 in, 1 out]
                          }
                          frame True {
                          }
                        }
                        n173 = Concatenate Strings(w7971, "ST201_R.BMP" ("字符串")) -> (w7989:string)
                        n174 = Build Path(base path=w7976, name or relative path="ST201_R" ("名称或相对路径")) -> (appended path=w7978:path)
                        n175 = call <vilib>:"Check if File or Folder Exists.vi"("error in (no error)"=w7977, "path"=w7978) -> ("error out"=w7979:errorcluster, "file or folder exists?"=w7980:bool)  [unwired: 7 in, 1 out]
                        n176 = case shown="假" w7980 {
                          tunnel: w7978 -> [w7997 w7999]
                          tunnel: [w7996 w7999] -> w7972
                          tunnel: w7979 -> [w7995 w7998]
                          tunnel: [w7994 w7998] -> _
                          frame False {
                            n177 = Create Folder(path (use dialog)=w7997, error in=w7995) -> (created path=w7996:path, error out=w7994:errorcluster)  [unwired: 1 in, 1 out]
                          }
                          frame True {
                          }
                        }
                        n178 = Build Path(base path=w7972, name or relative path=w7989) -> (appended path=w7970:path)
                        n179 = call "文件路径.vi"("文件路径"=w7970, "文件格式"=".BMP") -> ("新路径"=w7969:path)  [unwired: 9 in]
                        n180 = invoke on="ST201_R曲线" class="XYGraph (严格)" method="Export Image"(error in=w7992, "FileType"=enum32{"BMP", "EPS", "EMF", "PICT"}."BMP" ("文件类型"), "Target"=enum32{"File", "Clipboard"}."File" ("目标"), "Path"=w7969, "HideGrid"=FALSE ("隐藏网格"), "Overwrite"=TRUE ("隐藏网格")) -> (error out=w7974:errorcluster)  [unwired: 2 in, 7 out]
                        n181 = Move(source path=w7973, error in=w7974, 9:TRUE ("覆盖(F)"), 10:w7972) -> (error out=w7982:errorcluster)  [unwired: 1 in, 2 out]
                      }
                      frame #4 {
                        n182 = Tick Count (ms)() -> (millisecond timer value=w8008:u32)
                        n183 = Subtract(x=w8008, y=w8007) -> (x-y=→"画曲线T-201 2":u32)
                      }
                    }
                  }
                }
              }
              frame #2 {
                n184 = call "检查曲线文件.vi"("Folder Path"=path "D:/op201" ("路径")) -> ("Error Out"=w8011:errorcluster, "Exit?"=w8013:bool, "曲线文件路径"=w8012:path)  [unwired: 7 in, 1 out]
                "OP201文件?" <- w8013
                n185 = case shown="真" w8013 {
                  tunnel: w8012 -> [_ w8018]
                  tunnel: w8011 -> [w8014 w8017]
                  tunnel: [w8014 w8016] -> _
                  frame False {
                  }
                  frame True {
                    n186 = flat-sequence {
                      tunnel: [w8021] -> w8019
                      tunnel: w8018 -> [w8020]
                      tunnel: w8017 -> [w8022]
                      tunnel: [w8020] -> w8015
                      tunnel: w8019 -> [w8048]
                      tunnel: [w8038] -> w8016
                      tunnel: w8015 -> [w8029]
                      frame #0 {
                        n187 = call "EXCEL 画曲线.vi"("错误输入（无错误）"=w8022, "路径"=w8020) -> ("error IO"=w8021:errorcluster, "XY图"=→"ST201_L曲线":cluster{"X":dbl, "Y":dbl}[])  [unwired: 6 in, 2 out]
                      }
                      frame #1 {
                        n188 = local read "201二维码"() -> (w8027:string)
                        n189 = call "图片保存.vi"("一维码"=w8027) -> ("dup path"=w8039:path)  [unwired: 9 in, 1 out]
                        n190 = Build Path(base path=w8039, name or relative path=w8027) -> (appended path=w8040:path)
                        n191 = call <vilib>:"Check if File or Folder Exists.vi"("path"=w8040) -> ("error out"=w8042:errorcluster, "file or folder exists?"=w8041:bool)  [unwired: 8 in, 1 out]
                        n192 = case shown="假" w8041 {
                          tunnel: w8040 -> [w8059 w8061]
                          tunnel: [w8058 w8061] -> w8032
                          tunnel: w8042 -> [w8057 w8060]
                          tunnel: [w8056 w8060] -> w8033
                          frame False {
                            n193 = Create Folder(path (use dialog)=w8059, error in=w8057) -> (created path=w8058:path, error out=w8056:errorcluster)  [unwired: 1 in, 1 out]
                          }
                          frame True {
                          }
                        }
                        n194 = Concatenate Strings(w8027, "ST201_L.BMP" ("字符串")) -> (w8045:string)
                        n195 = Build Path(base path=w8032, name or relative path="ST201_L" ("名称或相对路径")) -> (appended path=w8034:path)
                        n196 = call <vilib>:"Check if File or Folder Exists.vi"("error in (no error)"=w8033, "path"=w8034) -> ("error out"=w8035:errorcluster, "file or folder exists?"=w8036:bool)  [unwired: 7 in, 1 out]
                        n197 = case shown="假" w8036 {
                          tunnel: w8034 -> [w8053 w8055]
                          tunnel: [w8052 w8055] -> w8028
                          tunnel: w8035 -> [w8051 w8054]
                          tunnel: [w8050 w8054] -> _
                          frame False {
                            n198 = Create Folder(path (use dialog)=w8053, error in=w8051) -> (created path=w8052:path, error out=w8050:errorcluster)  [unwired: 1 in, 1 out]
                          }
                          frame True {
                          }
                        }
                        n199 = Build Path(base path=w8028, name or relative path=w8045) -> (appended path=w8026:path)
                        n200 = call "文件路径.vi"("文件路径"=w8026, "文件格式"=".BMP") -> ("新路径"=w8025:path)  [unwired: 9 in]
                        n201 = invoke on="ST201_L曲线" class="XYGraph (严格)" method="Export Image"(error in=w8048, "FileType"=enum32{"BMP", "EPS", "EMF", "PICT"}."BMP" ("文件类型"), "Target"=enum32{"File", "Clipboard"}."File" ("目标"), "Path"=w8025, "HideGrid"=FALSE ("隐藏网格"), "Overwrite"=TRUE ("隐藏网格")) -> (error out=w8030:errorcluster)  [unwired: 2 in, 7 out]
                        n202 = Move(source path=w8029, error in=w8030, 9:TRUE ("覆盖(F)"), 10:w8028) -> (error out=w8038:errorcluster)  [unwired: 1 in, 2 out]
                      }
                    }
                  }
                }
              }
              frame #3 {
                n203 = local write "ST201文件移动中"(FALSE ("ST201文件移动中")) -> ()
              }
            }
            n204 = case shown="错误" w7927 {
              frame No Error {
                n205 = local write "201数据回复写入"(TRUE ("201数据回复写入")) -> ()
                n206 = local write "数据保存请求回复201"("1" ("数据保存请求回复201")) -> ()
              }
              frame Error {
                n207 = local write "201数据回复写入"(TRUE ("201数据回复写入")) -> ()
                n208 = local write "数据保存请求回复201"("2" ("数据保存请求回复201")) -> ()
                n209 = property on="错误信息" class="LstBox (严格)"() -> ("Item Names"=w8071:string[])  [unwired: 2 in, 2 out]
                n210 = Format Date/Time String(time format string (%c)="%Y-%m-%d %H:%M:%S" ("时间格式字符串(%c)")) -> (date/time string=w8073:string)  [unwired: 2 in]
                n211 = Concatenate Strings(w8073, "  " ("字符串"), "ST201 画曲线错误") -> (w8069:string)
                n212 = Insert Into Array(array=w8071, index=0 ("索引"), new element=w8069) -> (w8068:string[])
                n213 = property on="错误信息" class="LstBox (严格)"("Item Names"=w8068) -> ()  [unwired: 2 in, 2 out]
              }
            }
            "ST201画曲线" <- FALSE ("ST20画曲线")
          }
          event "ST202画曲线": Value Change {
            n214 = event-data() -> ()  [unwired: 1 in, 3 out]
            n215 = call "检查曲线文件.vi"("Folder Path"=path "D:/op202" ("路径")) -> ("Error Out"=w8076:errorcluster, "Exit?"=w8078:bool, "曲线文件路径"=w8077:path)  [unwired: 7 in, 1 out]
            n216 = case shown="真" w8078 {
              tunnel: w8077 -> [_ w8097]
              tunnel: w8076 -> [w8093 w8096]
              tunnel: [w8093 w8095] -> w8075
              frame False {
              }
              frame True {
                n217 = flat-sequence {
                  tunnel: [w8101] -> w8098
                  tunnel: w8097 -> [w8100]
                  tunnel: w8096 -> [w8102]
                  tunnel: [w8100] -> w8094
                  tunnel: w8098 -> [w8108]
                  tunnel: [w8122] -> w8095
                  tunnel: w8094 -> [w8114]
                  frame #0 {
                    n218 = call "EXCEL 画曲线.vi"("错误输入（无错误）"=w8102, "路径"=w8100) -> ("error IO"=w8101:errorcluster, "XY图"=→"ST202曲线":cluster{"X":dbl, "Y":dbl}[])  [unwired: 6 in, 2 out]
                  }
                  frame #1 {
                    n219 = local read "202二维码"() -> (w8110:string)
                    n220 = call "图片保存.vi"("一维码"=w8110) -> ("dup path"=w8123:path)  [unwired: 9 in, 1 out]
                    n221 = Build Path(base path=w8123, name or relative path=w8110) -> (appended path=w8124:path)
                    n222 = call <vilib>:"Check if File or Folder Exists.vi"("path"=w8124) -> ("error out"=w8126:errorcluster, "file or folder exists?"=w8125:bool)  [unwired: 8 in, 1 out]
                    n223 = case shown="假" w8125 {
                      tunnel: w8124 -> [w8138 w8140]
                      tunnel: [w8137 w8140] -> w8116
                      tunnel: w8126 -> [w8136 w8139]
                      tunnel: [w8135 w8139] -> w8117
                      frame False {
                        n224 = Create Folder(path (use dialog)=w8138, error in=w8136) -> (created path=w8137:path, error out=w8135:errorcluster)  [unwired: 1 in, 1 out]
                      }
                      frame True {
                      }
                    }
                    n225 = Concatenate Strings(w8110, "ST202.BMP" ("字符串")) -> (w8127:string)
                    n226 = Build Path(base path=w8116, name or relative path="ST202" ("名称或相对路径")) -> (appended path=w8118:path)
                    n227 = call <vilib>:"Check if File or Folder Exists.vi"("error in (no error)"=w8117, "path"=w8118) -> ("error out"=w8119:errorcluster, "file or folder exists?"=w8120:bool)  [unwired: 7 in, 1 out]
                    n228 = case shown="假" w8120 {
                      tunnel: w8118 -> [w8132 w8134]
                      tunnel: [w8131 w8134] -> w8113
                      tunnel: w8119 -> [w8130 w8133]
                      tunnel: [w8129 w8133] -> _
                      frame False {
                        n229 = Create Folder(path (use dialog)=w8132, error in=w8130) -> (created path=w8131:path, error out=w8129:errorcluster)  [unwired: 1 in, 1 out]
                      }
                      frame True {
                      }
                    }
                    n230 = Build Path(base path=w8113, name or relative path=w8127) -> (appended path=w8112:path)
                    n231 = call "文件路径.vi"("文件路径"=w8112, "文件格式"=".BMP") -> ("新路径"=w8104:path)  [unwired: 9 in]
                    n232 = invoke on="ST202曲线" class="XYGraph (严格)" method="Export Image"(error in=w8108, "FileType"=enum32{"BMP", "EPS", "EMF", "PICT"}."BMP" ("文件类型"), "Target"=enum32{"File", "Clipboard"}."File" ("目标"), "Path"=w8104, "HideGrid"=FALSE ("隐藏网格"), "Overwrite"=TRUE ("隐藏网格")) -> (error out=w8107:errorcluster)  [unwired: 2 in, 7 out]
                    n233 = Move(source path=w8114, error in=w8107, 9:TRUE ("覆盖(F)"), 10:w8113) -> (error out=w8122:errorcluster)  [unwired: 1 in, 2 out]
                  }
                }
              }
            }
            n234 = case shown="无错误" w8075 {
              frame No Error {
                n235 = local write "数据保存请求回复202"("1" ("数据保存请求回复202")) -> ()
                n236 = local write "202数据回复写入"(TRUE ("202数据回复写入")) -> ()
              }
              frame Error {
                n237 = local write "数据保存请求回复202"("2" ("数据保存请求回复202")) -> ()
                n238 = local write "202数据回复写入"(TRUE ("202数据回复写入")) -> ()
                n239 = property on="错误信息" class="LstBox (严格)"() -> ("Item Names"=w8089:string[])  [unwired: 2 in, 2 out]
                n240 = Format Date/Time String(time format string (%c)="%Y-%m-%d %H:%M:%S" ("时间格式字符串(%c)")) -> (date/time string=w8091:string)  [unwired: 2 in]
                n241 = Concatenate Strings(w8091, "  " ("字符串"), "ST202 画曲线错误") -> (w8087:string)
                n242 = Insert Into Array(array=w8089, index=0 ("索引"), new element=w8087) -> (w8086:string[])
                n243 = property on="错误信息" class="LstBox (严格)"("Item Names"=w8086) -> ()  [unwired: 2 in, 2 out]
              }
            }
            "ST202画曲线" <- FALSE ("ST202画曲线")
          }
          event "ST502画曲线": Value Change {
            n244 = event-data() -> ()  [unwired: 1 in, 3 out]
            n245 = stacked-sequence {
              tunnel: [w8144 _] -> w8141
              frame #0 {
                n246 = call "检查曲线文件.vi"("Folder Path"=path "D:/op50" ("路径")) -> ("Error Out"=w8145:errorcluster, "Exit?"=w8147:bool, "曲线文件路径"=w8146:path)  [unwired: 7 in, 1 out]
                n247 = case shown="真" w8147 {
                  tunnel: w8146 -> [_ w8153]
                  tunnel: w8145 -> [w8149 w8152]
                  tunnel: [w8149 w8151] -> w8144
                  frame False {
                  }
                  frame True {
                    n248 = flat-sequence {
                      tunnel: [w8156] -> w8154
                      tunnel: w8153 -> [w8155]
                      tunnel: w8152 -> [w8157]
                      tunnel: [w8155] -> w8150
                      tunnel: w8154 -> [w8183]
                      tunnel: [w8173] -> w8151
                      tunnel: w8150 -> [w8164]
                      frame #0 {
                        n249 = call "EXCEL 画曲线.vi"("错误输入（无错误）"=w8157, "路径"=w8155) -> ("error IO"=w8156:errorcluster, "XY图"=→"ST50_R曲线":cluster{"X":dbl, "Y":dbl}[])  [unwired: 6 in, 2 out]
                      }
                      frame #1 {
                        n250 = local read "502二维码"() -> (w8159:string)
                        n251 = call "图片保存.vi"("一维码"=w8159) -> ("dup path"=w8174:path)  [unwired: 9 in, 1 out]
                        n252 = Build Path(base path=w8174, name or relative path=w8159) -> (appended path=w8175:path)
                        n253 = call <vilib>:"Check if File or Folder Exists.vi"("path"=w8175) -> ("error out"=w8177:errorcluster, "file or folder exists?"=w8176:bool)  [unwired: 8 in, 1 out]
                        n254 = case shown="假" w8176 {
                          tunnel: w8175 -> [w8194 w8196]
                          tunnel: [w8193 w8196] -> w8167
                          tunnel: w8177 -> [w8192 w8195]
                          tunnel: [w8191 w8195] -> w8168
                          frame False {
                            n255 = Create Folder(path (use dialog)=w8194, error in=w8192) -> (created path=w8193:path, error out=w8191:errorcluster)  [unwired: 1 in, 1 out]
                          }
                          frame True {
                          }
                        }
                        n256 = Concatenate Strings(w8159, "ST50_R.BMP" ("字符串")) -> (w8180:string)
                        n257 = Build Path(base path=w8167, name or relative path="ST50_R" ("名称或相对路径")) -> (appended path=w8169:path)
                        n258 = call <vilib>:"Check if File or Folder Exists.vi"("error in (no error)"=w8168, "path"=w8169) -> ("error out"=w8170:errorcluster, "file or folder exists?"=w8171:bool)  [unwired: 7 in, 1 out]
                        n259 = case shown="假" w8171 {
                          tunnel: w8169 -> [w8188 w8190]
                          tunnel: [w8187 w8190] -> w8163
                          tunnel: w8170 -> [w8186 w8189]
                          tunnel: [w8185 w8189] -> _
                          frame False {
                            n260 = Create Folder(path (use dialog)=w8188, error in=w8186) -> (created path=w8187:path, error out=w8185:errorcluster)  [unwired: 1 in, 1 out]
                          }
                          frame True {
                          }
                        }
                        n261 = Build Path(base path=w8163, name or relative path=w8180) -> (appended path=w8162:path)
                        n262 = call "文件路径.vi"("文件路径"=w8162, "文件格式"=".BMP") -> ("新路径"=w8161:path)  [unwired: 9 in]
                        n263 = invoke on="ST50_R曲线" class="XYGraph (严格)" method="Export Image"(error in=w8183, "FileType"=enum32{"BMP", "EPS", "EMF", "PICT"}."BMP" ("文件类型"), "Target"=enum32{"File", "Clipboard"}."File" ("目标"), "Path"=w8161, "HideGrid"=FALSE ("隐藏网格"), "Overwrite"=TRUE ("隐藏网格")) -> (error out=w8165:errorcluster)  [unwired: 2 in, 7 out]
                        n264 = Move(source path=w8164, error in=w8165, 9:TRUE ("覆盖(F)"), 10:w8163) -> (error out=w8173:errorcluster)  [unwired: 1 in, 2 out]
                      }
                    }
                  }
                }
              }
              frame #1 {
                n265 = call "检查曲线文件.vi"("Folder Path"=path "D:/op50" ("路径")) -> ("Error Out"=w8198:errorcluster, "Exit?"=w8200:bool, "曲线文件路径"=w8199:path)  [unwired: 7 in, 1 out]
                n266 = case shown="真" w8200 {
                  tunnel: w8199 -> [_ w8205]
                  tunnel: w8198 -> [w8201 w8204]
                  tunnel: [w8201 w8203] -> _
                  frame False {
                  }
                  frame True {
                    n267 = flat-sequence {
                      tunnel: [w8208] -> w8206
                      tunnel: w8205 -> [w8207]
                      tunnel: w8204 -> [w8209]
                      tunnel: [w8207] -> w8202
                      tunnel: w8206 -> [w8235]
                      tunnel: [w8225] -> w8203
                      tunnel: w8202 -> [w8216]
                      frame #0 {
                        n268 = call "EXCEL 画曲线.vi"("错误输入（无错误）"=w8209, "路径"=w8207) -> ("error IO"=w8208:errorcluster, "XY图"=→"ST50_L曲线":cluster{"X":dbl, "Y":dbl}[])  [unwired: 6 in, 2 out]
                      }
                      frame #1 {
                        n269 = local read "502二维码"() -> (w8211:string)
                        n270 = call "图片保存.vi"("一维码"=w8211) -> ("dup path"=w8226:path)  [unwired: 9 in, 1 out]
                        n271 = Build Path(base path=w8226, name or relative path=w8211) -> (appended path=w8227:path)
                        n272 = call <vilib>:"Check if File or Folder Exists.vi"("path"=w8227) -> ("error out"=w8229:errorcluster, "file or folder exists?"=w8228:bool)  [unwired: 8 in, 1 out]
                        n273 = case shown="假" w8228 {
                          tunnel: w8227 -> [w8246 w8248]
                          tunnel: [w8245 w8248] -> w8219
                          tunnel: w8229 -> [w8244 w8247]
                          tunnel: [w8243 w8247] -> w8220
                          frame False {
                            n274 = Create Folder(path (use dialog)=w8246, error in=w8244) -> (created path=w8245:path, error out=w8243:errorcluster)  [unwired: 1 in, 1 out]
                          }
                          frame True {
                          }
                        }
                        n275 = Concatenate Strings(w8211, "ST50_L.BMP" ("字符串")) -> (w8232:string)
                        n276 = Build Path(base path=w8219, name or relative path="ST50_L" ("名称或相对路径")) -> (appended path=w8221:path)
                        n277 = call <vilib>:"Check if File or Folder Exists.vi"("error in (no error)"=w8220, "path"=w8221) -> ("error out"=w8222:errorcluster, "file or folder exists?"=w8223:bool)  [unwired: 7 in, 1 out]
                        n278 = case shown="假" w8223 {
                          tunnel: w8221 -> [w8240 w8242]
                          tunnel: [w8239 w8242] -> w8215
                          tunnel: w8222 -> [w8238 w8241]
                          tunnel: [w8237 w8241] -> _
                          frame False {
                            n279 = Create Folder(path (use dialog)=w8240, error in=w8238) -> (created path=w8239:path, error out=w8237:errorcluster)  [unwired: 1 in, 1 out]
                          }
                          frame True {
                          }
                        }
                        n280 = Build Path(base path=w8215, name or relative path=w8232) -> (appended path=w8214:path)
                        n281 = call "文件路径.vi"("文件路径"=w8214, "文件格式"=".BMP") -> ("新路径"=w8213:path)  [unwired: 9 in]
                        n282 = invoke on="ST50_L曲线" class="XYGraph (严格)" method="Export Image"(error in=w8235, "FileType"=enum32{"BMP", "EPS", "EMF", "PICT"}."BMP" ("文件类型"), "Target"=enum32{"File", "Clipboard"}."File" ("目标"), "Path"=w8213, "HideGrid"=FALSE ("隐藏网格"), "Overwrite"=TRUE ("隐藏网格")) -> (error out=w8217:errorcluster)  [unwired: 2 in, 7 out]
                        n283 = Move(source path=w8216, error in=w8217, 9:TRUE ("覆盖(F)"), 10:w8215) -> (error out=w8225:errorcluster)  [unwired: 1 in, 2 out]
                      }
                    }
                  }
                }
              }
            }
            n284 = case shown="无错误" w8141 {
              frame No Error {
                n285 = local write "数据保存请求回复502"("1" ("数据保存请求回复502")) -> ()
                n286 = local write "502数据回复输入"(TRUE ("502数据回复输入")) -> ()
              }
              frame Error {
                n287 = local write "数据保存请求回复502"("2" ("数据保存请求回复502")) -> ()
                n288 = local write "502数据回复输入"(TRUE ("502数据回复输入")) -> ()
                n289 = property on="错误信息" class="LstBox (严格)"() -> ("Item Names"=w8257:string[])  [unwired: 2 in, 2 out]
                n290 = Format Date/Time String(time format string (%c)="%Y-%m-%d %H:%M:%S" ("时间格式字符串(%c)")) -> (date/time string=w8259:string)  [unwired: 2 in]
                n291 = Concatenate Strings(w8259, "  " ("字符串"), "ST50 画曲线错误") -> (w8255:string)
                n292 = Insert Into Array(array=w8257, index=0 ("索引"), new element=w8255) -> (w8254:string[])
                n293 = property on="错误信息" class="LstBox (严格)"("Item Names"=w8254) -> ()  [unwired: 2 in, 2 out]
              }
            }
            "ST502画曲线" <- FALSE ("ST30画曲线 (事件)")
          }
          event "ST70画曲线": Value Change {
            n294 = event-data() -> ()  [unwired: 1 in, 3 out]
            n295 = stacked-sequence {
              tunnel: [_ w8325] -> w8261
              frame #0 {
                n296 = call "检查曲线文件.vi"("Folder Path"=path "D:/op70" ("路径")) -> ("Error Out"=w8263:errorcluster, "Exit?"=w8265:bool, "曲线文件路径"=w8264:path)  [unwired: 7 in, 1 out]
